vi "acc_master.vi"   [LabVIEW 2015]
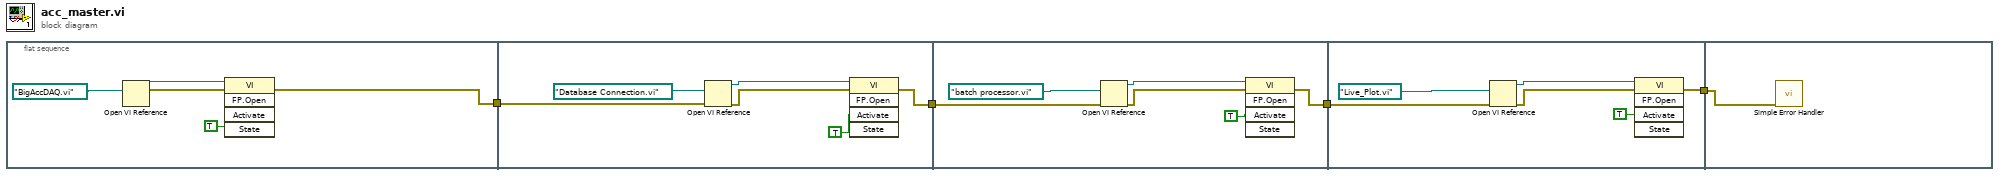
[diagram p0: block diagram]
diagram:
  n1 = flat-sequence {
    tunnel: [w5] -> w4
    tunnel: w4 -> [w11]
    tunnel: [w10] -> w3
    tunnel: w3 -> [w17]
    tunnel: [w16] -> w2
    tunnel: w2 -> [w23]
    tunnel: [w22] -> w1
    tunnel: w1 -> [w28]
    frame #0 {
      n2 = Open VI Reference(vi path=path "BigAccDAQ.vi") -> (vi reference=w8:refnum<vi>, error out=w7:errorcluster)  [unwired: 5 in]
      n3 = invoke class="VI" method="FP.Open"(reference=w8, error in=w7, "Activate"=TRUE ("Activate?")) -> (error out=w5:errorcluster)  [unwired: 2 in, 4 out]
    }
    frame #1 {
      n4 = Open VI Reference(vi path=path "Database Connection.vi", error in (no error)=w11) -> (vi reference=w13:refnum<vi>, error out=w14:errorcluster)  [unwired: 4 in]
      n5 = invoke class="VI" method="FP.Open"(reference=w13, error in=w14, "Activate"=TRUE ("Activate?")) -> (error out=w10:errorcluster)  [unwired: 2 in, 4 out]
    }
    frame #2 {
      n6 = Open VI Reference(vi path=path "batch processor.vi", error in (no error)=w17) -> (vi reference=w19:refnum<vi>, error out=w20:errorcluster)  [unwired: 4 in]
      n7 = invoke class="VI" method="FP.Open"(reference=w19, error in=w20, "Activate"=TRUE ("Activate?")) -> (error out=w16:errorcluster)  [unwired: 2 in, 4 out]
    }
    frame #3 {
      n8 = Open VI Reference(vi path=path "Live_Plot.vi", error in (no error)=w23) -> (vi reference=w25:refnum<vi>, error out=w26:errorcluster)  [unwired: 4 in]
      n9 = invoke class="VI" method="FP.Open"(reference=w25, error in=w26, "Activate"=TRUE ("Activate?")) -> (error out=w22:errorcluster)  [unwired: 2 in, 4 out]
    }
    frame #4 {
      n10 = call <vilib>:"Simple Error Handler.vi"("error in (no error)"=w28) -> ()  [unwired: 4 in, 5 out]
    }
  }
